vi "G4SubTemplate_Singleton_5x6x5_Init.vi"(0 "reference in":refnum<class "G4SubTemplate_Singleton_5x6x5.lvclass"> caption="This control should only be used when\na sub class is inheriting this class", 11 "error in (no error)":errorcluster) -> (4 "reference out":refnum<class "G4SubTemplate_Singleton_5x6x5.lvclass"> caption="This indicator should only be used when\na sub class is inheriting this class", 15 "error out":errorcluster)   [LabVIEW 2014, in "G4SubTemplate_Singleton_5x6x5.lvclass"]
uses:
  <resource>/Framework/Providers/Open_GDS/ClassProviders/Provider_EndevoGOOP400/Templates/G4SubTemplate_Singleton_5x6x5/G4SubTemplate_Singleton_5x6x5.lvclass
  <resource>/Framework/Providers/Open_GDS/ClassProviders/Provider_EndevoGOOP400/Templates/G4BaseTemplate_Singleton_5x6x5/G4BaseTemplate_Singleton_5x6x5.lvclass
panel:
  # "sub single 5x"
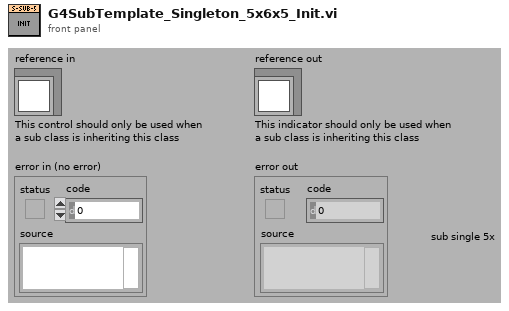
[diagram p1: front panel]
types:
  T1 = typedef "G4SubTemplate_Singleton_5x6x5.lvclass/ObjectAttributes.ctl" = cluster{"Attribute1":dbl}
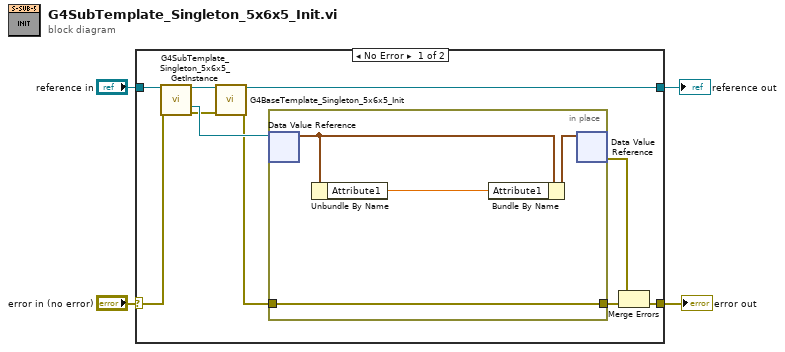
[diagram p0: block diagram]
diagram:
  n1 = case shown="No Error" "error in (no error)" {
    selector: "error in (no error)" -> [w11 w20]
    tunnel: [w12 w20] -> w3
    tunnel: "reference in" -> [w8 w19]
    tunnel: [w7 w19] -> w1
    frame No Error {
      n2 = call <resource>:"G4SubTemplate_Singleton_5x6x5_GetInstance.vi"("reference in"=w8, "error in (no error)"=w11) -> ("reference out"=w9:refnum<class "G4SubTemplate_Singleton_5x6x5.lvclass">, "DVRRefOut"=w14:refnum<data-value>, "error out"=w10:errorcluster)  [unwired: 9 in, 2 out]
      n3 = call <resource>:"G4BaseTemplate_Singleton_5x6x5_Init.vi"("reference in"=w9, "error in (no error)"=w10) -> ("reference out"=w7:refnum<class "G4SubTemplate_Singleton_5x6x5.lvclass">, "error out"=w6:errorcluster)  [unwired: 12 in]
      n4 = in-place {
        in-place-border: w6 -> [w15]
        in-place-border: [w15] -> w5
        n5 = in-place-dvr #1(w14) -> (w17:T1)  [unwired: 1 out]
        n6 = Unbundle By Name(w17) -> ("Attribute1"=w16:dbl)
        n7 = Bundle By Name(cluster=w17, "Attribute1"=w16) -> (w18:T1)
        n8 = in-place-dvr #1(w18) -> (w13:errorcluster)  [unwired: 1 out]
      }
      n9 = Merge Errors(w13, w5) -> (w12:errorcluster)
    }
    frame Error {
    }
  }
  "error out" <- w3
  "reference out" <- w1
